vi "Memory.Pointer.Get Address.vi"(8 "error in (no error)":errorcluster, 11 "Pointer in":refnum<class "Memory.Pointer.lvclass">) -> (0 "error out":errorcluster, 2 "address":u64 format="%016x", 3 "Pointer out":refnum<class "Memory.Pointer.lvclass">)   [LabVIEW 2016, in "LabVIEW Memory Manager.lvlib" / "Memory.Pointer.lvclass"]
uses:
  Memory.Pointer.lvclass
  Memory.Pointer.lvclass/Memory.Pointer.ctl
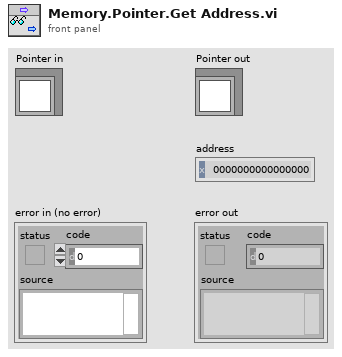
[diagram p1: front panel]
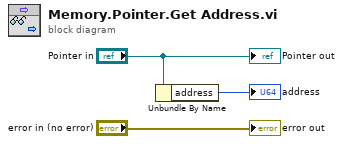
[diagram p0: block diagram]
diagram:
  n1 = Unbundle By Name("Pointer in") -> ("address"=→"address":u64)
  "error out" <- "error in (no error)"
  "Pointer out" <- "Pointer in"
